vi "test validation.vi"() -> ()   [LabVIEW 2013, in "NISE_CEF_Tests.lvlib"]
uses:
  Trunk/CEF_TreeControl/serializable configuration/NISE_CEF_serializable configuration.lvclass
  NISE_CEF_Tests.lvlib
panel:
  out "no error":errorcluster
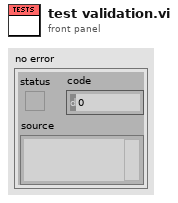
[diagram p1: front panel]
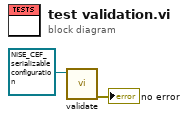
[diagram p0: block diagram]
diagram:
  n1 = call-dynamic "validate.vi"("configuration in"=refnum<class "NISE_CEF_serializable configuration.lvclass"> refnum ("configuration")) -> ("error out"=→"no error":errorcluster)  [unwired: 9 in, 1 out]
